vi "Stop Core.vi"(10 "final error code":i32, 11 "Debug Monitor in":refnum<class "Debug Monitor.lvclass">) -> (3 "Debug Monitor out":refnum<class "Debug Monitor.lvclass">)   [LabVIEW 2017, in "Debug Monitor.lvclass"]
doc: "(<B>Filename</B>: Actor Framework.lvlib:Actor.lvclass:Stop Core.vi)\n\nDefines what the actor does before it stops. Use the <B>final error code</B> input to determine whether the actor shut down in response to an error.\n\nBy default, this method does nothing. A descendant class may override it to define behavior, such as shutting down any processes the actor initiated in its override of the Actor Core method."
uses:
  Debug Monitor.lvclass
  Debug Monitor.lvclass/Debug Monitor.ctl
  Source/Actor Monitor/Actor Monitor/Actor Monitor.lvclass
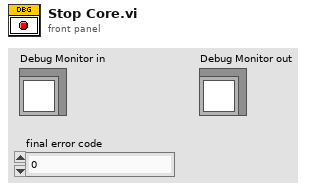
[diagram p1: front panel]
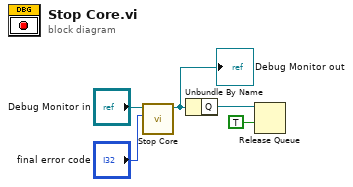
[diagram p0: block diagram]
diagram:
  n1 = call-parent "Stop Core.vi"("final error code"="final error code", "Actor in"="Debug Monitor in") -> ("Actor out"=w3:refnum<class "Debug Monitor.lvclass">)  [unwired: 9 in]
  "Debug Monitor out" <- w3
  n2 = Unbundle By Name(w3) -> ("Q"=w2:refnum<queue>)
  n3 = Release Queue(queue=w2, force destroy? (F)=TRUE) -> ()  [unwired: 1 in, 3 out]
